vi "C_VI.vi"(10 "Internal C":refnum<vi>, 11 "Notifier in":refnum<notifier>) -> (3 "VI out":refnum<vi>)   [LabVIEW 2015]
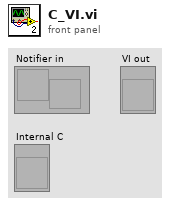
[diagram p1: front panel]
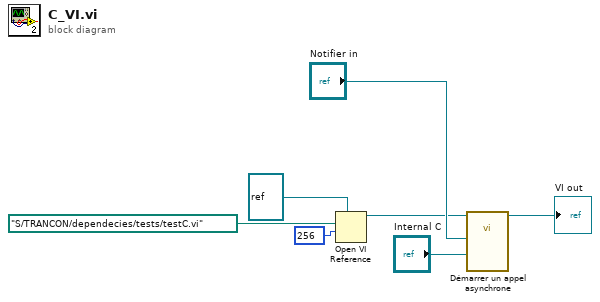
[diagram p0: block diagram]
diagram:
  n1 = Open VI Reference(type specifier VI Refnum (for type only)=refnum<vi> refnum ("spécificateur de type du refnum de VI (pour type seulement)"), vi path=path "S:/TRANCON/dependecies/tests/testC.vi" ("chemin du VI"), options=256) -> (vi reference=w4:refnum<vi>)  [unwired: 3 in, 1 out]
  n2 = call-by-ref "Démarrer un appel asynchrone"(reference=w4, "Internal C"="Internal C", "notifier out"="Notifier in") -> (reference out=→"VI out":refnum<vi>)  [unwired: 11 in, 1 out]
